vi "BK Precision 91xx (GPIB) Main Page.vi"(8 "error in (no error)":errorcluster, 11 "Node Ptr":T2 format="%.0x") -> (0 "error out":errorcluster)   [LabVIEW 2009, in "BK Precision 91xx (GPIB) Custom Device.lvlib"]
uses:
  BK Precision 91xx (GPIB) Custom Device.lvlib
  <vilib>/NI VeriStand/Custom Device API/Custom Device Item Ref.ctl
  Serial Config.ctl
  Global Strings.vi
  <vilib>/NI VeriStand/Custom Device API/Get Item Property (Variant).vi
  <vilib>/NI VeriStand/Custom Device API/Get Item Property (Boolean).vi
  <vilib>/NI VeriStand/Custom Device API/Get Item Property (U16).vi
  <vilib>/NI VeriStand/Custom Device API/Get Item Property (String).vi
  <vilib>/NI VeriStand/Custom Device API/Get Item Property (Double).vi
  <vilib>/NI VeriStand/Custom Device API/Set Item Property (String).vi
  <vilib>/NI VeriStand/Custom Device API/Set Item Property (Boolean).vi
  <vilib>/NI VeriStand/Custom Device API/Set Item Property (Double).vi
  <vilib>/NI VeriStand/Custom Device API/Set Item Property (U16).vi
  <vilib>/NI VeriStand/Custom Device API/Set Item Property (Variant).vi
  <vilib>/NI VeriStand/Custom Device API/Custom Device API.lvlib
panel:
  in  "Serial Configuration":T1={"Baud Rate"=9600, "Parity"=0, "Data Bits"=8, "Stop Bits"=10} {"Baud Rate" items=["1200"=1200, "2400"=2400, "4800"=4800, "9600"=9600]; "Parity" items=["None", "Odd", "Even"]; "Data Bits" items=["7"=7, "8"=8]; "Stop Bits" items=["1.0"=10]}
  in  "Perform ID Query?":bool=TRUE
  in  "Loop rate (ms)":u16
  in  "Voltage Limit":dbl(slide)=20.0 min=1.0 max=60.0 scale=1.0..35.0 scale format="%#.6g"
  in  "Enable OVP":bool=TRUE
  in  "VISA resource name":string
  in  "Header":cluster{"Section Name":string}={"Section Name"="BK Precision 91xx Item Settings"}
  in  "Description":string
  in  "Name":string
  in  "Delete":bool
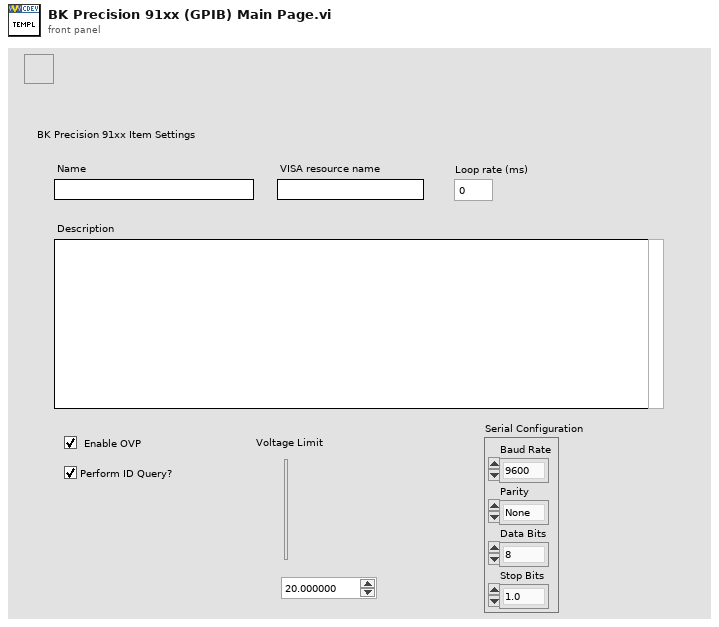
[diagram p1: front panel]
types:
  T1 = typedef "BK Precision 91xx (GPIB) Custom Device.lvlib/Serial Config.ctl" = cluster{"Baud Rate":u32, "Parity":u16, "Data Bits":u16, "Stop Bits":u16}
  T2 = typedef "Custom Device API.lvlib/Custom Device Item Ref.ctl" = u64
  T3 = typedef "Custom Device API.lvlib/Custom Device Item Info.ctl" = cluster{"Name":string, "Is Channel":bool, "GUID":string}
  T4 = typedef "Custom Device API.lvlib/Custom Device Commands.ctl" = enum16{"Default", "Item renamed", "Shutdown"}
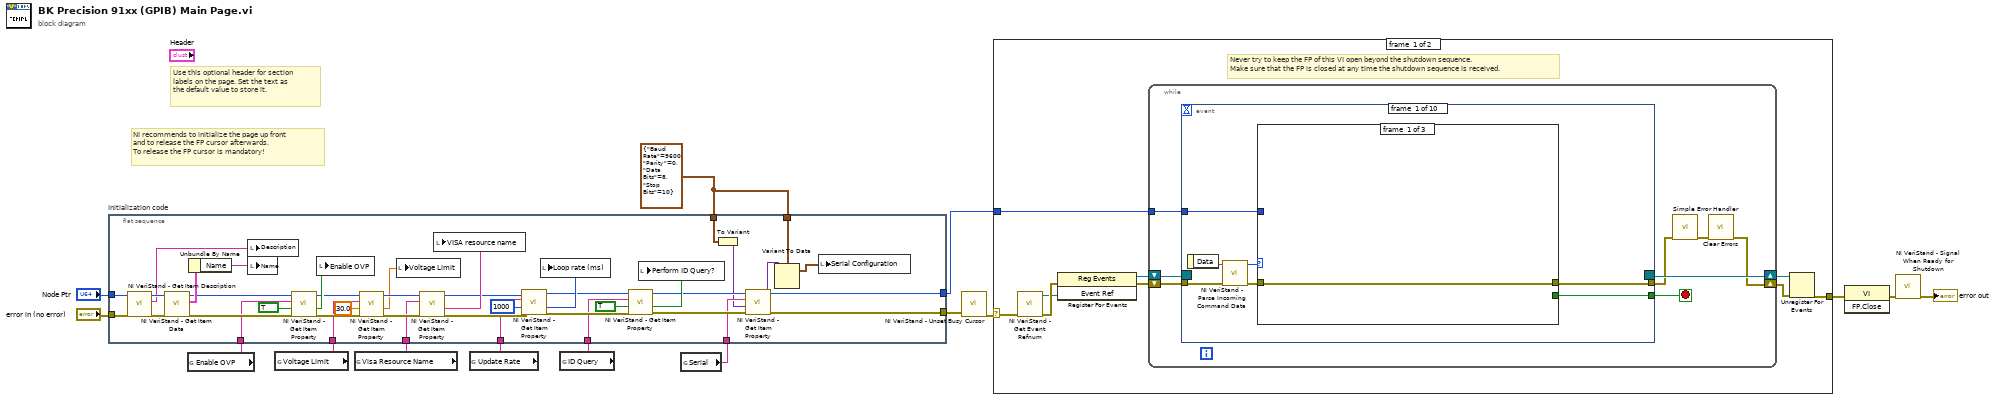
[diagram p0: block diagram]
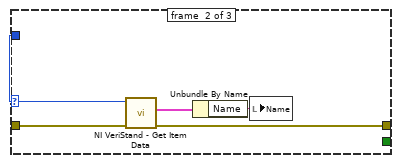
[diagram p2: hidden frame]
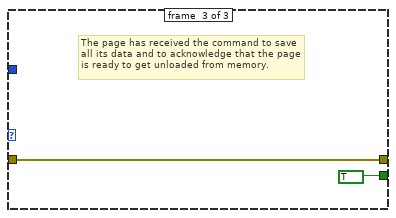
[diagram p3: hidden frame]
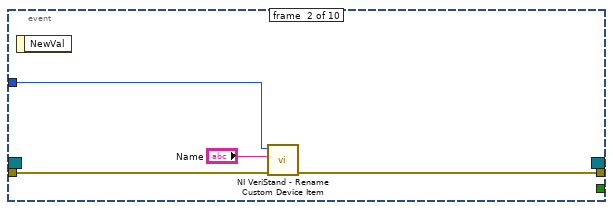
[diagram p4: hidden frame]
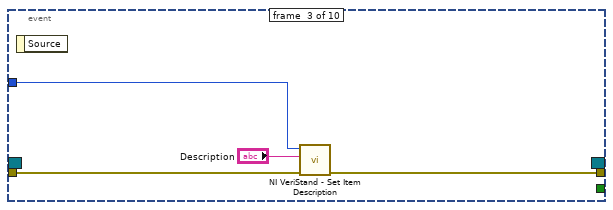
[diagram p5: hidden frame]
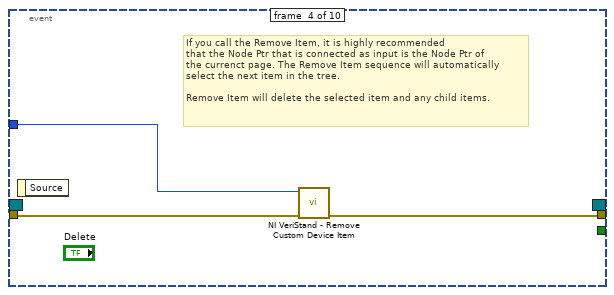
[diagram p6: hidden frame]
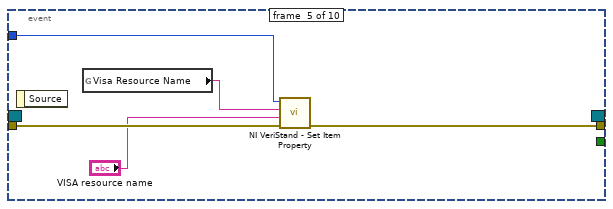
[diagram p7: hidden frame]
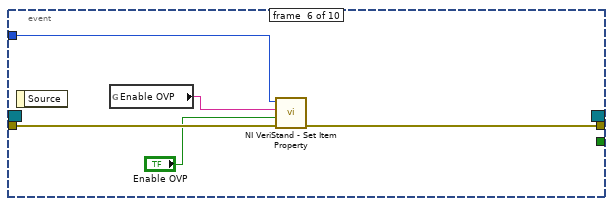
[diagram p8: hidden frame]
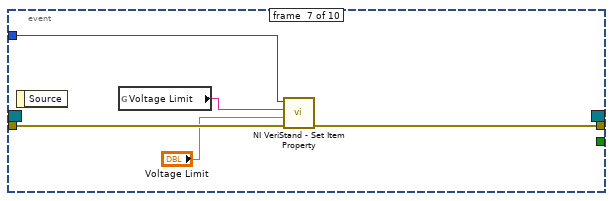
[diagram p9: hidden frame]
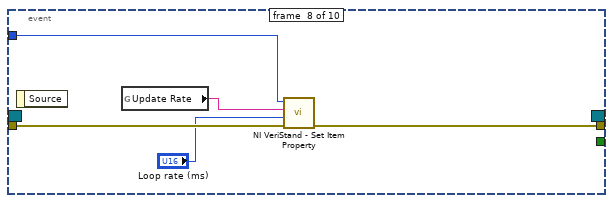
[diagram p10: hidden frame]
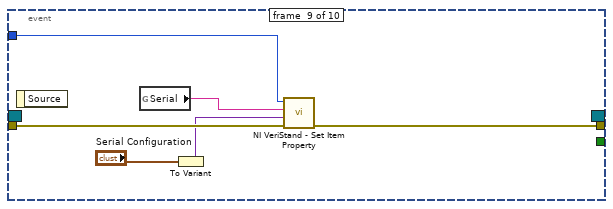
[diagram p11: hidden frame]
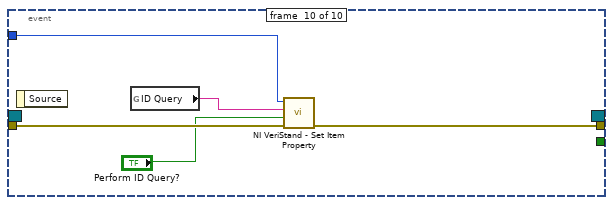
[diagram p12: hidden frame]
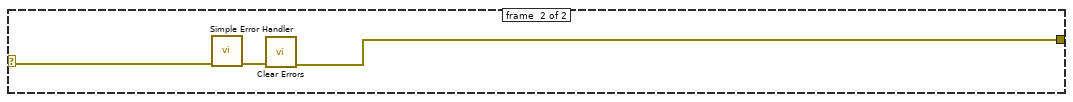
[diagram p13: hidden frame]
diagram:
  w2 = T1 {"Baud Rate"=9600, "Parity"=0, "Data Bits"=8, "Stop Bits"=10} ("Serial Configuration")
  # "Use this optional header for section labels on the page. Set the text as the default value to store it."
  # "NI recommends to initialize the page up front\nand to release the FP cursor afterwards.\nTo release the FP cursor is mandatory!"
  n1 = flat-sequence "Initialization code" {
    tunnel: "error in (no error)" -> [w55]
    tunnel: "Node Ptr" -> [w54]
    tunnel: [w22] -> w9
    tunnel: w8 -> [w47]
    tunnel: w7 -> [w42]
    tunnel: w6 -> [w38]
    tunnel: w5 -> [w34]
    tunnel: w4 -> [w28]
    tunnel: w3 -> [w23]
    tunnel: w2 -> [w19]
    tunnel: w2 -> [w18]
    tunnel: [w16] -> w1
    frame #0 {
      n2 = call <vilib>:"NI VeriStand - Get Item Description.vi"("error in (no error)"=w55, "Item Ref in"=w54) -> ("error out"=w52:errorcluster, "Description"=w53:string, "Item Ref out"=w56:T2)  [unwired: 7 out]
      n3 = call <vilib>:"NI VeriStand - Get Item Data.vi"("error in (no error)"=w52, "Item Ref in"=w56) -> ("error out"=w49:errorcluster, "Item Info"=w51:T3, "Item Ref out"=w48:T2)  [unwired: 7 out]
      n4 = Unbundle By Name(w51) -> ("Name"=w50:string)
      n5 = local write "Description"(w53) -> ()
      n6 = local write "Name"(w50) -> ()
      n7 = call-poly <vilib>:"NI VeriStand - Get Item Property.vi"("error in (no error)"=w49, "Default Value"=TRUE, "Property Name"=w47, "Item Ref in"=w48) -> ("error out"=w44:errorcluster, "Value"=w45:bool, "Item Ref out"=w43:T2)  [unwired: 4 in, 1 out]
      n8 = local write "Enable OVP"(w45) -> ()
      n9 = call-poly <vilib>:"NI VeriStand - Get Item Property.vi"("error in (no error)"=w44, "Default Value"=30.0, "Property Name"=w42, "Item Ref in"=w43) -> ("error out"=w40:errorcluster, "Value"=w37:dbl, "Item Ref out"=w39:T2)  [unwired: 4 in, 1 out]
      n10 = local write "Voltage Limit"(w37) -> ()
      n11 = call-poly <vilib>:"NI VeriStand - Get Item Property.vi"("error in (no error)"=w40, "Property Name"=w38, "Item Ref in"=w39) -> ("error out"=w35:errorcluster, "Value"=w36:string, "Item Ref out"=w33:T2)  [unwired: 5 in, 1 out]
      n12 = local write "VISA resource name"(w36) -> ()
      n13 = call-poly <vilib>:"NI VeriStand - Get Item Property.vi"("error in (no error)"=w35, "Default Value"=u16 1000, "Property Name"=w34, "Item Ref in"=w33) -> ("error out"=w30:errorcluster, "Value"=w31:u16, "Item Ref out"=w29:T2)  [unwired: 4 in, 1 out]
      n14 = local write "Loop rate (ms)"(w31) -> ()
      n15 = call-poly <vilib>:"NI VeriStand - Get Item Property.vi"("error in (no error)"=w30, "Default Value"=TRUE, "Property Name"=w28, "Item Ref in"=w29) -> ("error out"=w25:errorcluster, "Value"=w26:bool, "Item Ref out"=w24:T2)  [unwired: 4 in, 1 out]
      n16 = local write "Perform ID Query?"(w26) -> ()
      n17 = To Variant(anything=w19) -> (Variant=w20:variant)
      n18 = call-poly <vilib>:"NI VeriStand - Get Item Property.vi"("error in (no error)"=w25, "Default Value"=w20, "Property Name"=w23, "Item Ref in"=w24) -> ("error out"=w16:errorcluster, "Value"=w21:variant, "Item Ref out"=w22:T2)  [unwired: 4 in, 1 out]
      n19 = Variant To Data(Variant=w21, type=w18) -> (data=w17:T1)  [unwired: 1 in, 1 out]
      n20 = local write "Serial Configuration"(w17) -> ()
    }
  }
  n21 = global read "Global Strings.vi" "Enable OVP"() -> (w8:string)
  n22 = global read "Global Strings.vi" "Voltage Limit"() -> (w7:string)
  n23 = global read "Global Strings.vi" "Visa Resource Name"() -> (w6:string)
  n24 = global read "Global Strings.vi" "Update Rate"() -> (w5:string)
  n25 = global read "Global Strings.vi" "ID Query"() -> (w4:string)
  n26 = global read "Global Strings.vi" "Serial"() -> (w3:string)
  n27 = call <vilib>:"NI VeriStand - Unset Busy Cursor.vi"("error in (no error)"=w1) -> ("error out"=w11:errorcluster)  [unwired: 10 out]
  n28 = case shown="No Error" w11 {
    selector: w11 -> [w57 w133]
    tunnel: [w62 w131] -> w15
    tunnel: w9 -> [w58 _]
    frame #0 {
      # "Never try to keep the FP of this VI open beyond the shutdown sequence.\nMake sure that the FP is closed at any time the shutdown sequence is received."
      n29 = call <vilib>:"NI VeriStand - Get Event Refnum.vi"("error in (no error)"=w57) -> ("error out"=w65:errorcluster, "Event Ref"=w61:refnum<user-event>)  [unwired: 9 out]
      n30 = register-events(error in=w65, w61) -> (reference out=w59:refnum<event-registration>, error out=w60:errorcluster)  [unwired: 1 in]
      n31 = while {
        tunnel: w58 -> [w69]
        shift-right: [w66] -> w63
        shift-left: w60 -> [w72]
        shift-right: [w73] -> w64
        shift-left: w59 -> [w71]
        stop <- w70 stop-if-true
        n32 = event shown="[8] \"Serial Configuration\": Value Change" {
          selector: w71 -> [_ _ _ _ _ _ _ _ _ _]
          dyn-events: [_ _ _ _ _ _ _ _ _ _] -> w73
          timeout: _ -> [_ _ _ _ _ _ _ _ _ _]
          tunnel: w72 -> [w80 w92 w95 w99 w104 w109 w114 w119 w125 w130]
          tunnel: [w76 _ _ _ _ _ _ _ _ _] -> w70
          tunnel: [w75 w91 w94 w98 w103 w108 w113 w118 w124 w129] -> w68
          tunnel: w69 -> [w74 w90 w96 w97 w102 w107 w110 w116 w122 w127]
          event #0 {
            n33 = event-data() -> ("Data"=w79:string)  [unwired: 1 out]
            n34 = call <vilib>:"NI VeriStand - Parse Incoming Command Data.vi"("error in (no error)"=w80, "Data"=w79) -> ("error out"=w78:errorcluster, "Action"=w77:T4)  [unwired: 8 out]
            n35 = case shown="\"Item renamed\"" w77 {
              tunnel: w78 -> [w81 w86 w87]
              tunnel: [_ _ TRUE] -> w76
              tunnel: [w81 w83 w87] -> w75
              tunnel: w74 -> [_ w85 _]
              frame #0 {
              }
              frame #1 {
                n36 = call <vilib>:"NI VeriStand - Get Item Data.vi"("error in (no error)"=w86, "Item Ref in"=w85) -> ("error out"=w83:errorcluster, "Item Info"=w84:T3)  [unwired: 8 out]
                n37 = Unbundle By Name(w84) -> ("Name"=w82:string)
                n38 = local write "Name"(w82) -> ()
              }
              frame #2 {
                # "The page has received the command to save all its data and to acknowledge that the page is ready to get unloaded from memory."
              }
            }
          }
          event #1 {
            n39 = event-data() -> ()  [unwired: 2 out]
            n40 = call <vilib>:"NI VeriStand - Rename Custom Device Item.vi"("error in (no error)"=w92, "New Name"="Name", "Item Ref in"=w90) -> ("error out"=w91:errorcluster)  [unwired: 8 out]
          }
          event #2 {
            n41 = event-data() -> ()  [unwired: 2 out]
            n42 = call <vilib>:"NI VeriStand - Set Item Description.vi"("error in (no error)"=w95, "Description"="Description", "Item Ref in"=w96) -> ("error out"=w94:errorcluster)  [unwired: 8 out]
          }
          event #3 {
            # "If you call the Remove Item, it is highly recommended\nthat the Node Ptr that is connected as input is the Node Ptr of\nthe currenct page. The Remove Item sequence will automatically\nselect the next item in the tree.\n\nRemove Item will delete the selected item and any child items."
            n43 = event-data() -> ()  [unwired: 2 out]
            n44 = call <vilib>:"NI VeriStand - Remove Custom Device Item.vi"("error in (no error)"=w99, "Item Ref in"=w97) -> ("error out"=w98:errorcluster)  [unwired: 1 in, 8 out]
          }
          event #4 {
            n45 = event-data() -> ()  [unwired: 2 out]
            n46 = global read "Global Strings.vi" "Visa Resource Name"() -> (w101:string)
            n47 = call-poly <vilib>:"NI VeriStand - Set Item Property.vi"("error in (no error)"=w104, "Value"="VISA resource name", "Property Name"=w101, "Item Ref in"=w102) -> ("error out"=w103:errorcluster)  [unwired: 5 in, 2 out]
          }
          event #5 {
            n48 = event-data() -> ()  [unwired: 2 out]
            n49 = global read "Global Strings.vi" "Enable OVP"() -> (w106:string)
            n50 = call-poly <vilib>:"NI VeriStand - Set Item Property.vi"("error in (no error)"=w109, "Value"="Enable OVP", "Property Name"=w106, "Item Ref in"=w107) -> ("error out"=w108:errorcluster)  [unwired: 5 in, 2 out]
          }
          event #6 {
            n51 = event-data() -> ()  [unwired: 2 out]
            n52 = global read "Global Strings.vi" "Voltage Limit"() -> (w111:string)
            n53 = call-poly <vilib>:"NI VeriStand - Set Item Property.vi"("error in (no error)"=w114, "Value"="Voltage Limit", "Property Name"=w111, "Item Ref in"=w110) -> ("error out"=w113:errorcluster)  [unwired: 5 in, 2 out]
          }
          event #7 {
            n54 = event-data() -> ()  [unwired: 2 out]
            n55 = global read "Global Strings.vi" "Update Rate"() -> (w117:string)
            n56 = call-poly <vilib>:"NI VeriStand - Set Item Property.vi"("error in (no error)"=w119, "Value"="Loop rate (ms)", "Property Name"=w117, "Item Ref in"=w116) -> ("error out"=w118:errorcluster)  [unwired: 5 in, 2 out]
          }
          event #8 {
            n57 = event-data() -> ()  [unwired: 2 out]
            n58 = global read "Global Strings.vi" "Serial"() -> (w123:string)
            n59 = To Variant(anything="Serial Configuration") -> (Variant=w120:variant)
            n60 = call-poly <vilib>:"NI VeriStand - Set Item Property.vi"("error in (no error)"=w125, "Value"=w120, "Property Name"=w123, "Item Ref in"=w122) -> ("error out"=w124:errorcluster)  [unwired: 5 in, 2 out]
          }
          event #9 {
            n61 = event-data() -> ()  [unwired: 2 out]
            n62 = global read "Global Strings.vi" "ID Query"() -> (w128:string)
            n63 = call-poly <vilib>:"NI VeriStand - Set Item Property.vi"("error in (no error)"=w130, "Value"="Perform ID Query?", "Property Name"=w128, "Item Ref in"=w127) -> ("error out"=w129:errorcluster)  [unwired: 5 in, 2 out]
          }
        }
        n64 = call <vilib>:"Simple Error Handler.vi"("error in (no error)"=w68) -> ("error out"=w67:errorcluster)  [unwired: 1 in, 7 out]
        n65 = call <vilib>:"Clear Errors.vi"("error in (no error)"=w67) -> ("error out"=w66:errorcluster)  [unwired: 6 out]
      }
      n66 = Unregister For Events(event registration refnum=w64, error in=w63) -> (error out=w62:errorcluster)
    }
    frame #1 {
      n67 = call <vilib>:"Simple Error Handler.vi"("error in (no error)"=w133) -> ("error out"=w132:errorcluster)  [unwired: 1 in, 7 out]
      n68 = call <vilib>:"Clear Errors.vi"("error in (no error)"=w132) -> ("error out"=w131:errorcluster)  [unwired: 6 out]
    }
  }
  n69 = invoke class="VI" method="FP.Close"(error in=w15) -> (error out=w14:errorcluster)  [unwired: 2 in, 2 out]
  n70 = call <vilib>:"NI VeriStand - Signal When Ready for Shutdown.vi"("error in (no error)"=w14) -> ("error out"=→"error out":errorcluster)  [unwired: 10 out]
